vi "DataError Event Callback.vi"(4 "DataGridView in":refnum<class "DataGridView.lvclass">, 5 "Event Data":cluster{"sender":refnum<k24>, "e":refnum<k24>}, 6 "Control Ref":refnum<k24>, 7 "Event Common Data":T1) -> ()   [LabVIEW 2014, in "DataGrid.lvlib" / "DataGridView.lvclass"]
uses:
  DataGridView/DataGridView.lvclass
  System.Windows.Forms
  DataError/DataError.lvclass
  DataError/DataError.lvclass/DataError.ctl
  DataError/Write ColumnIndex.vi
  DataError/Write Context.vi
  DataError/Write Exception.vi
  DataError/Write RowIndex.vi
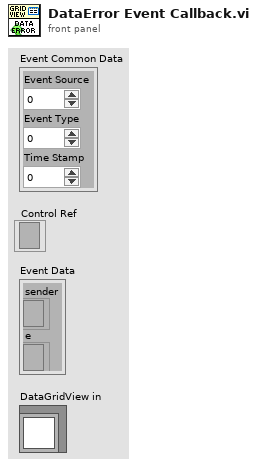
[diagram p1: front panel]
types:
  T1 = cluster{"Event Source":i32, "Event Type":u32, "Time Stamp":u32}
  T2 = cluster{"CellClicked":refnum<user-event>, "CellValue Changed":refnum<user-event>, "KeyDown":refnum<user-event>, "DataError":refnum<user-event>, "UserAddedRow":refnum<user-event>, "UserDeletedRow":refnum<user-event>}
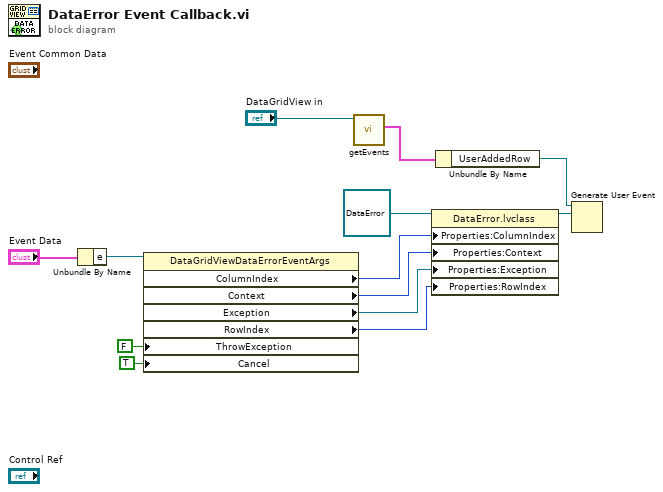
[diagram p0: block diagram]
diagram:
  n1 = Unbundle By Name("Event Data") -> ("e"=w12:refnum<k24>)
  n2 = property class="DataGridViewDataErrorEventArgs"(reference=w12, "ThrowException"=FALSE, "Cancel"=TRUE) -> ("ColumnIndex"=w5:i32, "Context"=w4:i32, "Exception"=w3:refnum<k24>, "RowIndex"=w2:i32)  [unwired: 1 in, 2 out]
  n3 = call "getEvents.vi"("DataGridView in"="DataGridView in") -> ("userEvents"=w10:T2)  [unwired: 8 in, 2 out]
  n4 = property class="DataError.lvclass"(reference=refnum<class "DataError.lvclass"> refnum ("DataGrid.lvlib:DataError.lvclass"), "Properties:ColumnIndex"=w5, "Properties:Context"=w4, "Properties:Exception"=w3, "Properties:RowIndex"=w2) -> (reference out=w8:refnum<class "DataError.lvclass">)  [unwired: 1 in, 1 out]
  n5 = Unbundle By Name(w10) -> ("UserAddedRow"=w9:refnum<user-event>)
  n6 = Generate User Event(user event=w9, event data cluster=w8) -> ()  [unwired: 2 in, 2 out]
